vi "Engine-SystemAI-Ch06.vi"(1 "dt [s]":sgl=1.0 format="%0.2f", 2 "AI06 [V]":sgl) -> (0 "AI06":T1)   [LabVIEW 2016, in "DSI-RT.lvlib"]
uses:
  DSI-RT.lvlib
  Shared/Typedefs/Engine-Channel.ctl
  <vilib>/Analysis/3filter.llb/Filter Passband Type.ctl
  <vilib>/addons/Software Calibration Management/xSCM/Controls/TBL1D.ctl
  <vilib>/addons/Software Calibration Management/xSCM/Controls/TLU1D.ctl
  <vilib>/addons/Software Calibration Management/xSCM/CalPoint.xnode
  <vilib>/ptbypt/NI_PtbyPt.lvlib
  <vilib>/Analysis/NI_AALBase.lvlib
  Shared/DSI-Shared.lvlib
  <vilib>/addons/Software Calibration Management/xSCM/ni_scm.dll
  <vilib>/addons/Software Calibration Management/xSCM/SCM-API.lvlib
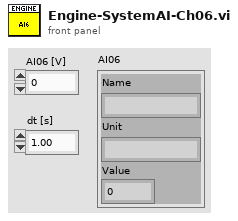
[diagram p1: front panel]
types:
  T1 = typedef "DSI-Shared.lvlib/Engine-Channel.ctl" = cluster{"Name":string, "Unit":string, "Value":sgl}
  T2 = typedef "NI_AALBase.lvlib/Filter Passband Type.ctl" = enum32{"Lowpass", "Highpass", "Bandpass", "Bandstop"}
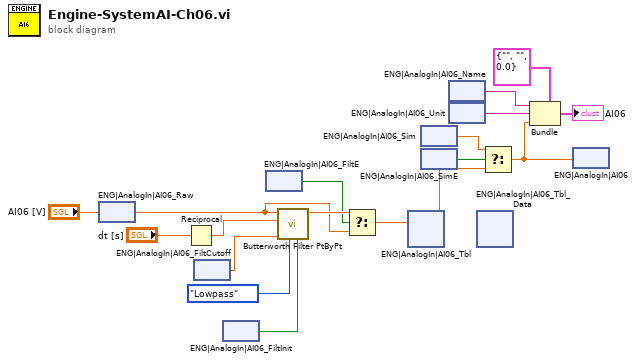
[diagram p0: block diagram]
diagram:
  n1 = xnode "ENG|AnalogIn|AI06_Raw"("Value"="AI06 [V]") -> ()
  n2 = Reciprocal(x="dt [s]") -> (1/x=w14:sgl)
  n3 = xnode "ENG|AnalogIn|AI06_FiltCutoff"() -> ("Value"=w12:sgl)
  n4 = xnode "ENG|AnalogIn|AI06_FiltInit"() -> ("Value"=w11:bool)
  n5 = xnode "ENG|AnalogIn|AI06_FiltE"() -> ("Value"=w8:bool)
  n6 = call <vilib>:"Butterworth Filter PtByPt.vi"("initialize"=w11, "filter type"=Filter_Passband_Type."Lowpass", "low cutoff freq: fl"=w12, "sampling freq: fs"=w14, "x"="AI06 [V]") -> ("Filtered x"=w10:dbl)  [unwired: 4 in, 1 out]
  n7 = Select(t=w10, s=w8, f="AI06 [V]") -> (s? t:f=w7:dbl)
  n8 = xnode "ENG|AnalogIn|AI06_Tbl"("X Index"=w7) -> ("Y"=w6:sgl)
  n9 = xnode "ENG|AnalogIn|AI06_Sim"() -> ("Value"=w16:sgl)
  n10 = xnode "ENG|AnalogIn|AI06_SimE"() -> ("Value"=w17:bool)
  n11 = xnode "ENG|AnalogIn|AI06_Name"() -> ("Value"=w4:string)
  n12 = xnode "ENG|AnalogIn|AI06_Unit"() -> ("Value"=w3:string)
  n13 = xnode "ENG|AnalogIn|AI06_Tbl_Data"() -> ()  [unwired: 1 out]
  n14 = Select(t=w16, s=w17, f=w6) -> (s? t:f=w1:sgl)
  n15 = Bundle(cluster=T1 {"Name"="", "Unit"="", "Value"=0.0} ("AI06"), "Name"=w4, "Unit"=w3, "Value"=w1) -> (→"AI06":T1)
  n16 = xnode "ENG|AnalogIn|AI06"("Value"=w1) -> ()
